vi "PipBoy_DestroyReferences.vi"(8 "error in (no error)":errorcluster, 10 "PipBoyData":T1) -> (0 "error out":errorcluster)   [LabVIEW 2014]
uses:
  ctls/PipBoy_PipBoyData.ctl
  ctls/PipBoy_ProcComm.ctl
  System.Windows.Forms
  ctls/PipBoy_PipBoyCommand.ctl
  ctls/PipBoy_Message.ctl
  modules/support/Message Queue/All Message Queues.ctl
  modules/support/Message Queue/Message Cluster.ctl
  ctls/PipBoy_FileConf.ctl
  ctls/PipBoy_PicComm.ctl
  ctls/PipBoy_GeneralParams.ctl
  ctls/PipBoy_Pages.ctl
  modules/support/User Event - Stop/User Event - Stop.lvlib
  modules/support/Message Queue/Message Queue.lvlib
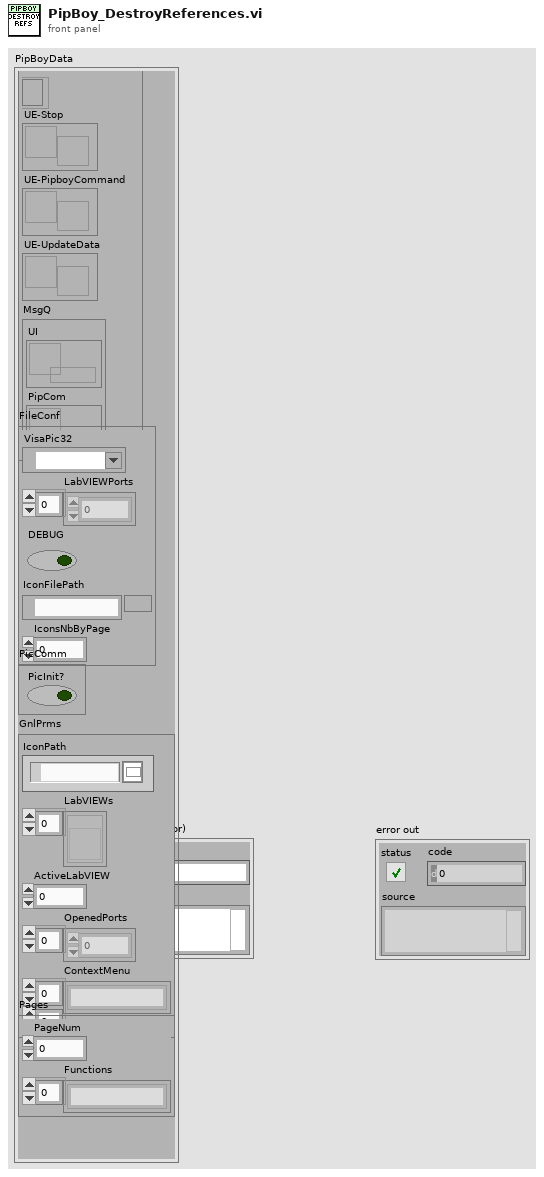
[diagram p1: front panel]
types:
  T1 = typedef "PipBoy_PipBoyData.ctl" = cluster{"ProcComm":T2, "FileConf":T4, "PicComm":T5, "GnlPrms":T6, "Pages":T7}
  T2 = typedef "PipBoy_ProcComm.ctl" = cluster{"NotifyIconRef":refnum<k24>, "UE-Stop":refnum<user-event>, "UE-PipboyCommand":refnum<user-event>, "UE-UpdateData":refnum<user-event>, "MsgQ":T3}
  T3 = typedef "Message Queue.lvlib/All Message Queues.ctl" = cluster{"UI":refnum<queue>, "PipCom":refnum<queue>}
  T4 = typedef "PipBoy_FileConf.ctl" = cluster{"VisaPic32":refnum<visa-resource-name>, "LabVIEWPorts":u16[], "DEBUG":bool, "IconFilePath":path, "IconsNbByPage":i32}
  T5 = typedef "PipBoy_PicComm.ctl" = cluster{"PicInit?":bool}
  T6 = typedef "PipBoy_GeneralParams.ctl" = cluster{"IconPath":path, "LabVIEWs":refnum<vi>[], "ActiveLabVIEW":i32, "OpenedPorts":u16[], "ContextMenu":string[][]}
  T7 = typedef "PipBoy_Pages.ctl" = cluster{"PageNum":i32, "Functions":string[]}
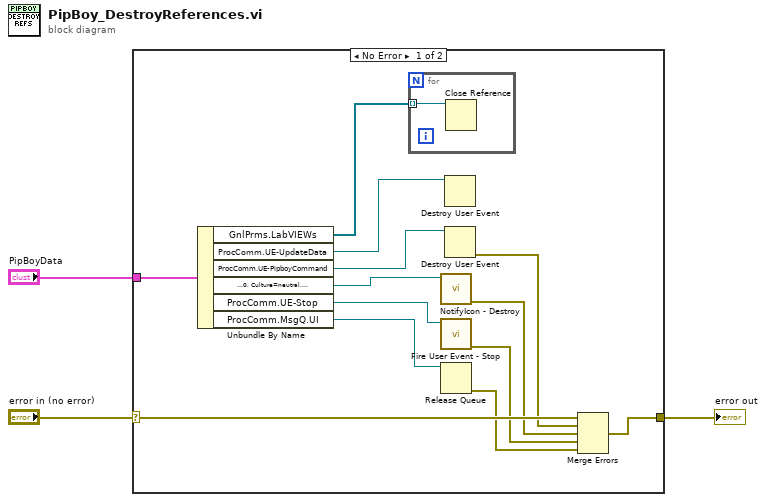
[diagram p0: block diagram]
diagram:
  n1 = case shown="No Error" "error in (no error)" {
    selector: "error in (no error)" -> [w11 w18]
    tunnel: [w12 w18] -> w2
    tunnel: "PipBoyData" -> [w13 _]
    frame No Error {
      n2 = Unbundle By Name(w13) -> ("GnlPrms.LabVIEWs"=w5:refnum<vi>[], "ProcComm.UE-UpdateData"=w4:refnum<user-event>, "ProcComm.UE-PipboyCommand"=w10:refnum<user-event>, "ProcComm.NotifyIconRef"=w14:refnum<k24>, "ProcComm.UE-Stop"=w15:refnum<user-event>, "ProcComm.MsgQ.UI"=w16:refnum<queue>)
      n3 = for {
        tunnel: w5 -> [w17] mode=indexing
        n4 = Close Reference(reference=w17) -> ()  [unwired: 1 in, 1 out]
      }
      n5 = call <userlib>:"NotifyIcon - Destroy.vi"("NotifyIcon reference"=w14) -> ("error out"=w7:errorcluster)  [unwired: 10 in]
      n6 = call "Fire User Event - Stop.vi"("User Event - Stop"=w15) -> ("error out"=w8:errorcluster)  [unwired: 10 in]
      n7 = Release Queue(queue=w16) -> (error out=w9:errorcluster)  [unwired: 2 in, 2 out]
      n8 = Destroy User Event(user event=w4) -> ()  [unwired: 1 in, 1 out]
      n9 = Destroy User Event(user event=w10) -> (error out=w6:errorcluster)  [unwired: 1 in]
      n10 = Merge Errors(w11, w6, w7, w8, w9) -> (w12:errorcluster)
    }
    frame Error {
    }
  }
  "error out" <- w2
